vi "Rescript Warning Dialog.vi"(8 "error in (no error)":errorcluster) -> (0 "error out":errorcluster, 1 "Cancelled?":bool)   [LabVIEW 2020, in "Message Rescripter.lvlib"]
uses:
  Message Rescripter.lvlib
  <resource>/dialog/lvconfig.llb/LV Config Write Boolean.vi
  <resource>/dialog/lvconfig.llb/LV Config Read Boolean.vi
panel:
  in  "Do not show this dialog again.":bool
  in  "Cancel Button":bool
  in  "Continue Button":bool
  # "You are about to rescript this message class.  If you continue, any custom code in your message class will be removed.  \n\nNational Instruments recommends that you NOT attempt to automatically rescript this message class if you have made any significant modifications to it.\n\nClick Continue to proceed with rescripting, or Cancel to abort the operation."
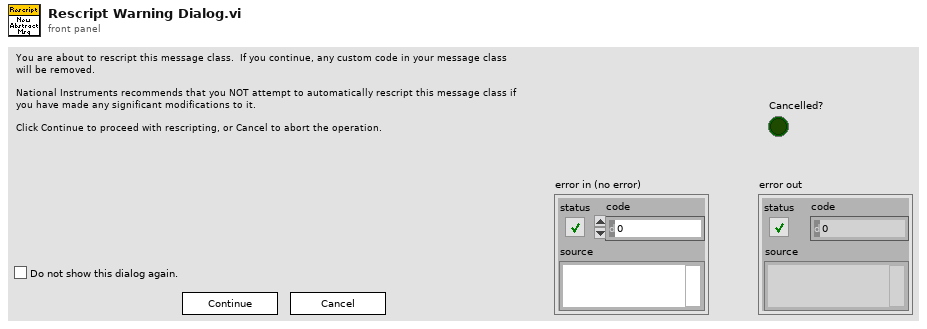
[diagram p1: front panel]
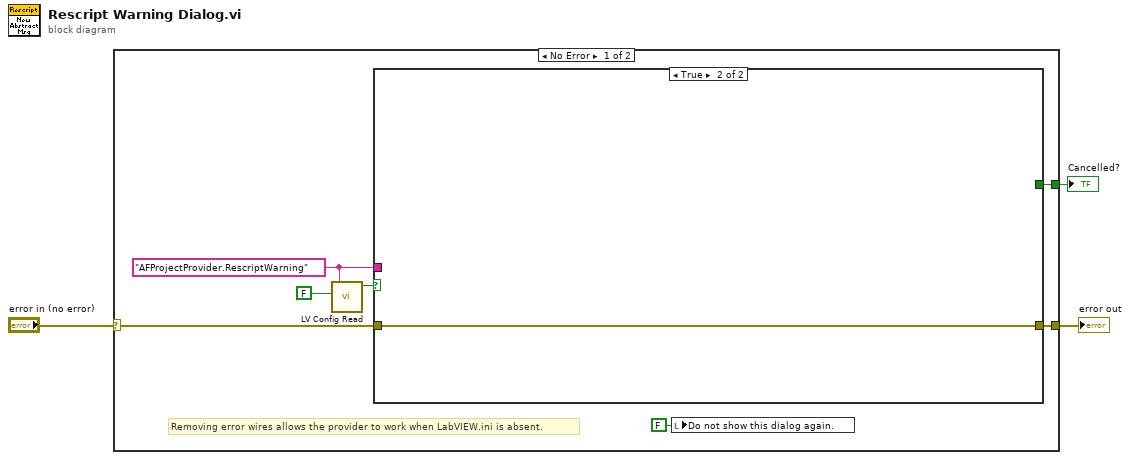
[diagram p0: block diagram]
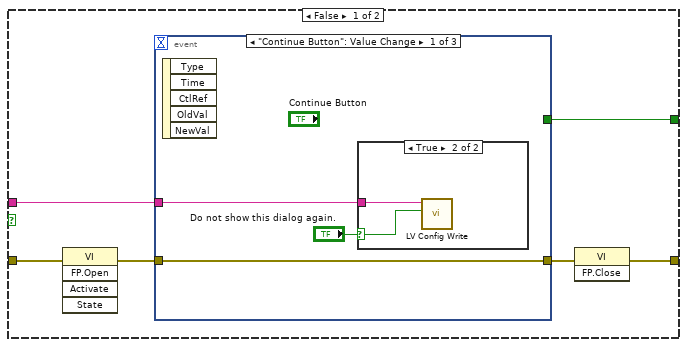
[diagram p2: hidden frame]
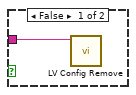
[diagram p3: hidden frame]
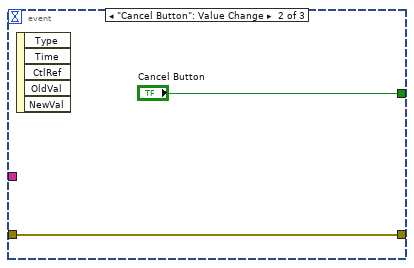
[diagram p4: hidden frame]
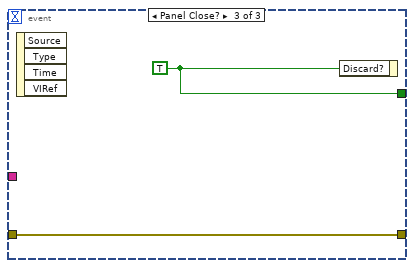
[diagram p5: hidden frame]
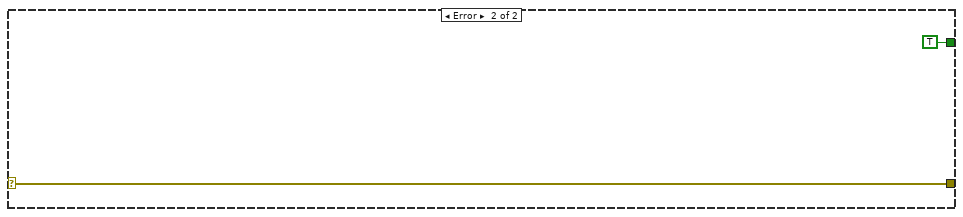
[diagram p6: hidden frame]
diagram:
  n1 = case shown="No Error" "error in (no error)" {
    selector: "error in (no error)" -> [w4 w28]
    tunnel: [w10 TRUE ("Discard?")] -> w3
    tunnel: [w6 w28] -> w1
    frame No Error {
      w7 = "AFProjectProvider.RescriptWarning" ("key")
      # "Removing error wires allows the provider to work when LabVIEW.ini is absent."
      n2 = call-poly <resource>:"LV Config Read.vi"("default value"=FALSE ("Use Reference Method"), "key"=w7) -> ("value"=w8:bool)  [unwired: 3 in, 2 out]
      n3 = case shown="True" w8 {
        tunnel: [w16 _] -> w10
        tunnel: w7 -> [w15 _]
        tunnel: w4 -> [w14 w27]
        tunnel: [w11 w27] -> w6
        frame False {
          n4 = invoke class="VI" method="FP.Open"(error in=w14) -> (error out=w13:errorcluster)  [unwired: 4 in, 4 out]
          n5 = event shown="[0] \"Continue Button\": Value Change" {
            selector: _ -> [_ _ _]
            dyn-events: _ -> [_ _ _]
            timeout: _ -> [_ _ _]
            tunnel: [_ "Cancel Button" w26] -> w16
            tunnel: w15 -> [w19 _ _]
            tunnel: w13 -> [w17 w23 w25]
            tunnel: [w17 w23 w25] -> w12
            event "Continue Button": Value Change {
              n6 = event-data() -> ()  [unwired: 1 in, 5 out]
              n7 = case shown="True" "Do not show this dialog again." {
                selector: "Do not show this dialog again." -> [_ w21]
                tunnel: w19 -> [w20 w22]
                frame False {
                  n8 = call <resource>:"LV Config Remove.vi"("key"=w20) -> ()  [unwired: 6 in, 1 out]
                }
                frame True {
                  n9 = call-poly <resource>:"LV Config Write.vi"("value"=w21, "key"=w22) -> ()  [unwired: 5 in, 1 out]
                }
              }
            }
            event "Cancel Button": Value Change {
              n10 = event-data() -> ()  [unwired: 1 in, 5 out]
            }
            event Panel Close? {
              w26 = TRUE ("Discard?")
              n11 = event-data() -> ()  [unwired: 1 in, 4 out]
              n12 = event-data("Discard?"=w26) -> ()  [unwired: 1 in, 1 out]
            }
          }
          n13 = invoke class="VI" method="FP.Close"(error in=w12) -> (error out=w11:errorcluster)  [unwired: 2 in, 2 out]
        }
        frame True {
        }
      }
      n14 = local write "Do not show this dialog again."(FALSE ("Don't show this dialog again.")) -> ()
    }
    frame Error {
    }
  }
  "Cancelled?" <- w3
  "error out" <- w1
